vi "rapportLivraison.vi"(10 "chemin de base":path, 11 "n° commande":string="6340/07-02.01.01") -> (0 "error IO":errorcluster, 3 "Titre fichier":string)   [LabVIEW 2020]
uses:
  Modules/Fonction Standard/Fichier ou dossier/Cluster des Chemins.ctl
panel:
  out "Texte fichier":string
  out "Tab cmde GPAO":string[][](array[string])=[["12-216C-04521", "EQIFIL ", "104mA    230ohm", "03104/08-05.01.01", "3", "221769", "EMAIL VOM 01.04.08  ", "BLATTY AG", "", "      ", "Fluid Automation Systems SA             ", "ALL", "0"], ["12-216C-04521", "EQIFIL ", "104mA    230ohm", "03128/08-01.01.01", "2", "226006", "RETURN FROM VIASYS2 ", "Fluid Automat. Systems GmbH", "", "      ", "Fluid Automation Systems SA             ", "ALL", "1"], ["12-216C-04521", "EQIFIL ", "104mA    230ohm", "03130/08-01.01.01", "1", "226005", "RETURN FROM VIASYS1 ", "Fluid Automat. Systems GmbH", "", "      ", "Fluid Automation Systems SA             ", "ALL", "1"], ["12-216C-04521", "EQIFIL ", "104mA    230ohm", "03365/08-01.01.01", "4", "225536", "SANS PAPIERS GE     ", "Fluid Automat. Systems GmbH", "", "      ", "Fluid Automation Systems SA             ", "ALL", "1"], ["12-216C-04521", "EQIFIL ", "104mA    230ohm", "03570/08-02.01.01", "100", "225052", "SANS PAPIERS        ", "IMI International Sp. z o.o.", "", "      ", "Fluid Automation Systems SA             ", "ANG", "1"], ["12-216C-04521", "EQIFIL ", "104mA    230ohm", "05066/08-01.01.01", "13", "225726", "120830              ", "Fluid Automat. Systems GmbH", "", "      ", "Fluid Automation Systems SA             ", "ALL", "1"], ["12-216C-04521", "EQIFIL ", "104mA    230ohm", "05067/08-01.01.01", "11", "225727", "120831              ", "Fluid Automat. Systems GmbH", "", "      ", "Fluid Automation Systems SA             ", "ALL", "1"]]
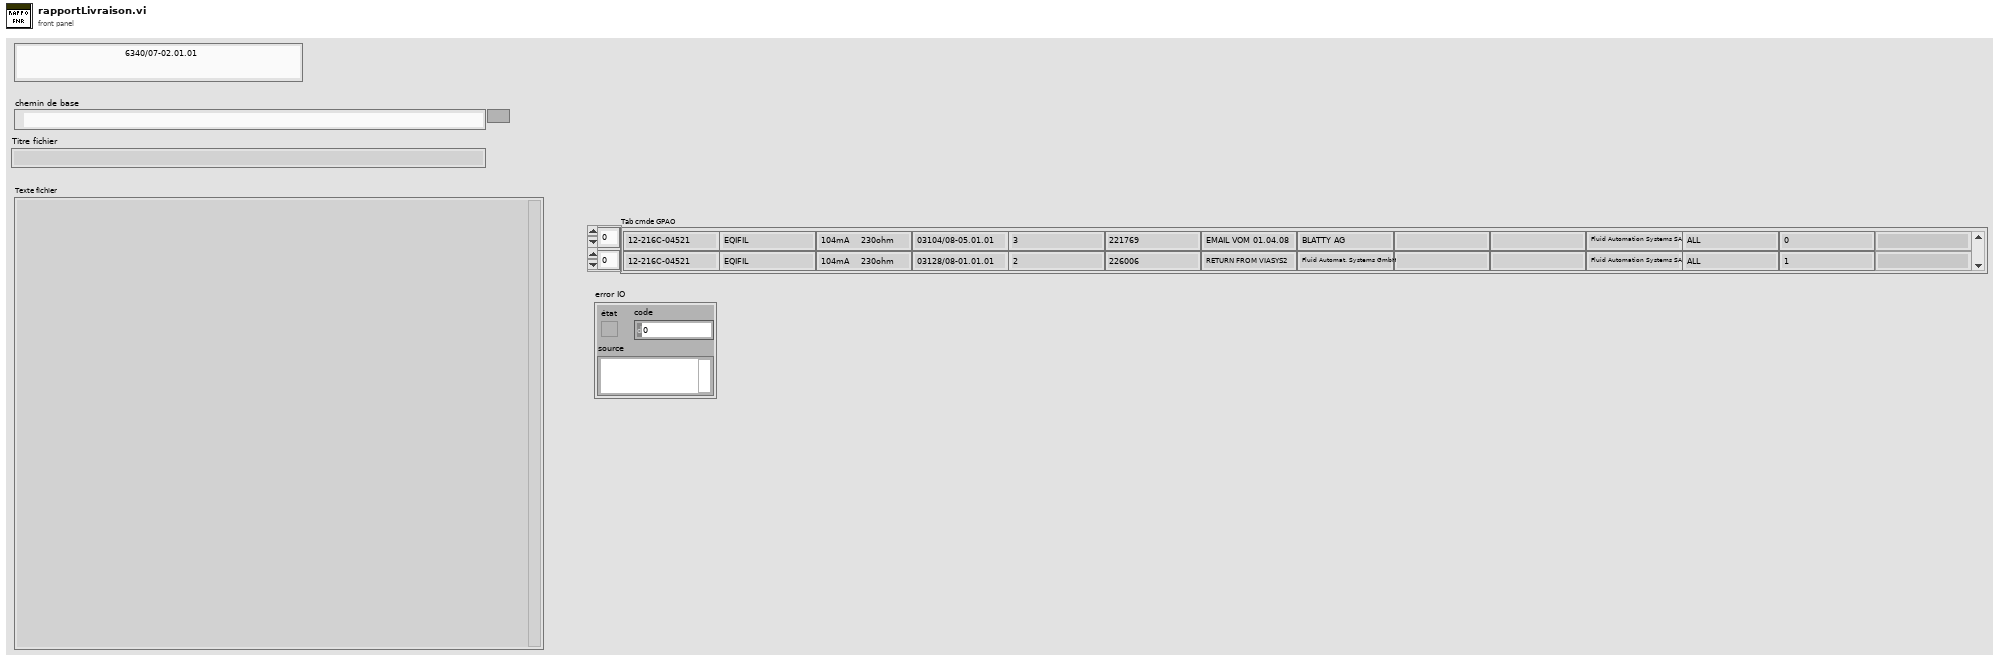
[diagram p1: front panel]
types:
  T1 = typedef "DATA commande.ctl" = cluster{"n°article FAS":string, "n° cmde FAS":string, "quantité cmde":string, "ID LIG cmde":string, "n° cmde client":string, "nom client":string, "n° article client":string, "indice revision client":string, "société de facturation":string, "langue a utiliser":string}
  T2 = typedef "Cluster des Chemins.ctl" = cluster{" Admin-réseau ":path, " XML-Réseau":path, " Résultat tests-Réseau":path, " Archive prôbleme-Réseau":path, " Archive Test  Local":path}
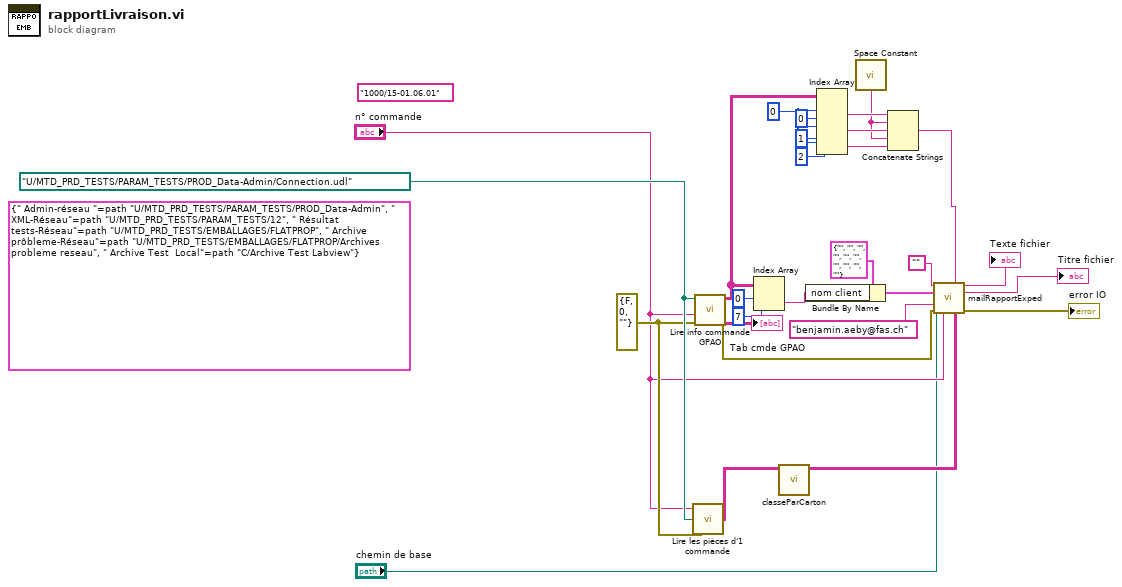
[diagram p0: block diagram]
diagram:
  w15 = 0 ("indice (ligne)")
  w18 = errorcluster {"status"=FALSE, "code"=0, "source"=""} ("error in (no error)")
  (unwired) "1000/15-01.06.01" ("n° commande")
  w19 = path "U:/MTD_PRD_TESTS/PARAM_TESTS/PROD_Data-Admin/Connection.udl" ("connection information")
  (unwired) T2 {" Admin-réseau "=path "U:/MTD_PRD_TESTS/PARAM_TESTS/PROD_Data-Admin", " XML-Réseau"=path "U:/MTD_PRD_TESTS/PARAM_TESTS/12", " Résultat tests-Réseau"=path "U:/MTD_PRD_TESTS/EMBALLAGES/FLATPROP", " Archive prôbleme-Réseau"=path "U:/MTD_PRD_TESTS/EMBALLAGES/FLATPROP/Archives probleme reseau", " Archive Test  Local"=path "C:/Archive Test Labview"} ("Chemins-News")
  n1 = call "Lire les pièces d'1 commande.vi"("n° commande"="n° commande", "connection information"=w19, "error in (no error)"=w18) -> ("Tableau"=w3:string[][])  [unwired: 4 out]
  n2 = call "Lire info commande GPAO.vi"("error in"=w18, "commande"="n° commande", "connection information"=w19) -> ("error out"=w21:errorcluster, "Tab cmde GPAO"=w16:string[][])  [unwired: 5 in, 2 out]
  "Tab cmde GPAO" <- w16
  n3 = Index Array(array=w16, index (row)=0 ("indice (ligne)"), index (col)=7 ("indice désactivé (col)")) -> (element=w24:string)
  n4 = call "classeParCarton.vi"("Tableau"=w3) -> ("triParCarton"=w2:string[][])  [unwired: 9 in, 1 out]
  n5 = Bundle By Name(cluster=T1 {"n°article FAS"="", "n° cmde FAS"="", "quantité cmde"="", "ID LIG cmde"="", "n° cmde client"="", "nom client"="", "n° article client"="", "indice revision client"="", "société de facturation"="", "langue a utiliser"=""} ("DATA cmde"), "nom client"=w24) -> (w25:T1)
  n6 = Index Array(array=w16, index (row) #1=w15, index (col) #1=0 ("indice désactivé (col)"), index (row) #2=w15, index (col) #2=1 ("indice désactivé (col)"), index (row) #3=w15, index (col) #3=2 ("indice désactivé (col)")) -> (element #1=w11:string, element #2=w10:string, element #3=w9:string)
  n7 = call <vilib>:"Space Constant.vi"() -> ("String"=w8:string)
  n8 = Concatenate Strings(w11, w8, w10, w8, w9) -> (w7:string)
  n9 = call "mailRapportExped.vi"("chaine valves"="", "produit"=w7, "DATA cmde"=w25, "chemin de base"="chemin de base", "Email Expédition"="benjamin.aeby@fas.ch", "error in (no error)"=w21, "n° cmde"="n° commande", "tab histo filtré\n par n° cmde"=w2) -> ("Texte fichier"=→"Texte fichier":string, "Titre fichier"=→"Titre fichier":string, "error out"=→"error IO":errorcluster)  [unwired: 5 in]
